vi "Suspend.vi"(8 "error in (no error)":errorcluster, 11 "Motor-GWInstek in":refnum<class "Motor-GWInstek.lvclass">) -> (0 "error out":errorcluster, 3 "Motor-GWInstek out":refnum<class "Motor-GWInstek.lvclass">)   [LabVIEW 2013, in "PowderDeposition.lvlib" / "Motor-GWInstek.lvclass"]
uses:
  Motor-GWInstek.lvclass
  Motor-GWInstek.lvclass/Motor-GWInstek.ctl
  Read Channel.vi
  <instrlib>/GPD-2303/GPD-2303.lvlib
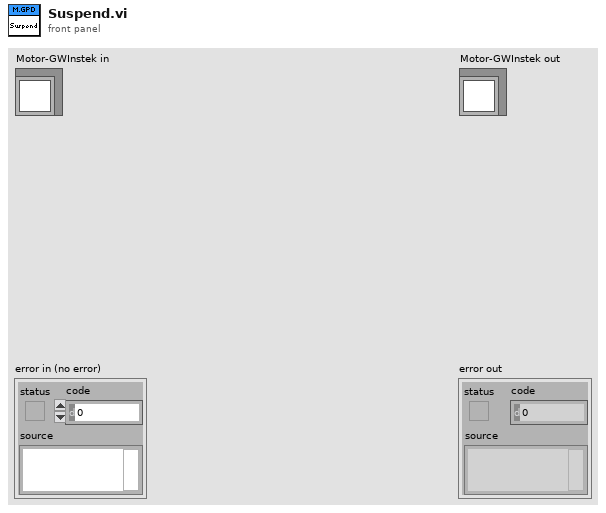
[diagram p1: front panel]
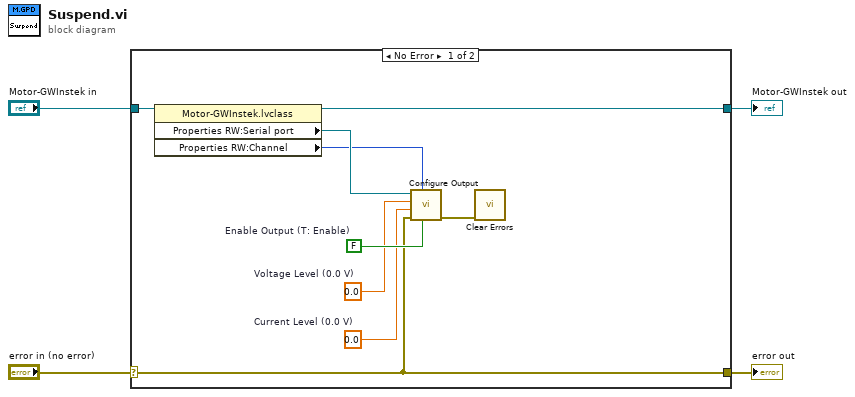
[diagram p0: block diagram]
diagram:
  n1 = case shown="No Error" "error in (no error)" {
    selector: "error in (no error)" -> [w8 w15]
    tunnel: [w8 w15] -> w3
    tunnel: [w12 w14] -> w1
    tunnel: "Motor-GWInstek in" -> [w13 w14]
    frame No Error {
      w9 = 0.0  # Current Level (0.0 V)
      w7 = 0.0  # Voltage Level (0.0 V)
      w10 = FALSE  # Enable Output (T: Enable)
      n2 = property class="Motor-GWInstek.lvclass"(reference=w13) -> (reference out=w12:refnum<class "Motor-GWInstek.lvclass">, "Properties RW:Serial port"=w11:refnum<visa-resource-name>, "Properties RW:Channel"=w6:i32)  [unwired: 1 in, 1 out]
      n3 = call <instrlib>:"Configure Output.vi"("Enable Output (T: Enable)"=w10, "Channel (1: Channel 1)"=w6, "error in (no error)"=w8, "Current Level (0.0 V)"=w9, "Voltage Level (0.0 V)"=w7, "VISA resource name"=w11) -> ("error out"=w5:errorcluster)  [unwired: 4 in, 1 out]
      n4 = call <vilib>:"Clear Errors.vi"("error in (no error)"=w5) -> ()  [unwired: 6 in, 1 out]
    }
    frame Error {
    }
  }
  "error out" <- w3
  "Motor-GWInstek out" <- w1
